vi "getStateValue.vi"(8 "error in (no error)":errorcluster, 11 "ScriptEvent in":refnum<class "ScriptEvent.lvclass">) -> (0 "error out":errorcluster, 2 "stateValue":string, 3 "ScriptEvent out":refnum<class "ScriptEvent.lvclass">)   [LabVIEW 2011, in "Tools.lvlib" / "Scripting.lvlib" / "ScriptEvent.lvclass"]
uses:
  ScriptEvent.lvclass
  ScriptEvent.lvclass/ScriptEvent.ctl
  DatabaseHelpers/Database Objects/Channel/Channel.lvclass
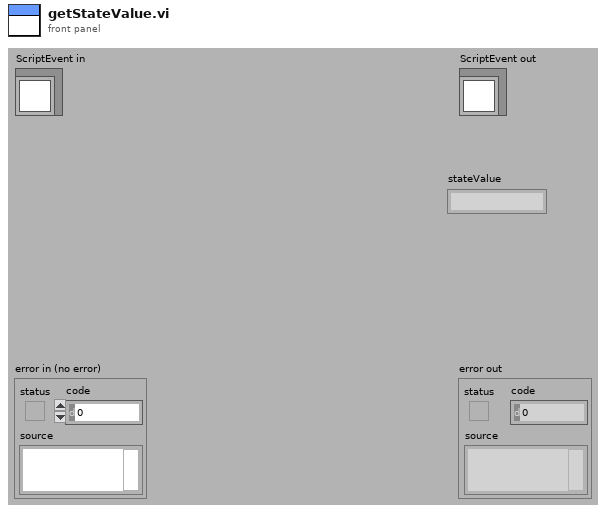
[diagram p1: front panel]
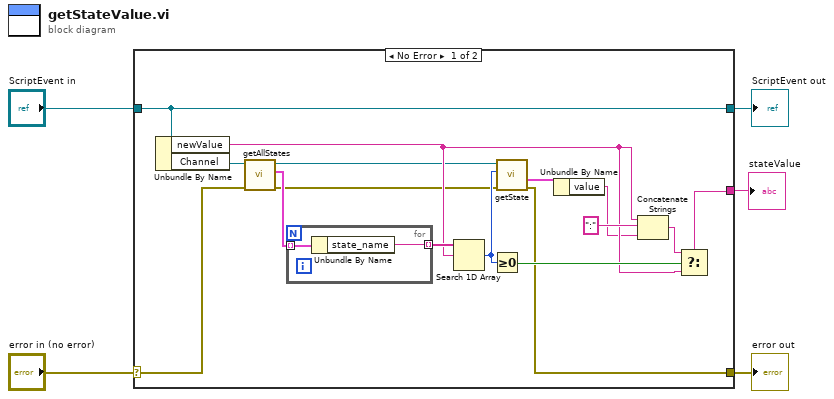
[diagram p0: block diagram]
diagram:
  n1 = case shown="No Error" "error in (no error)" {
    selector: "error in (no error)" -> [w10 w25]
    tunnel: [w6 w25] -> w4
    tunnel: [w21 w24] -> w2
    tunnel: "ScriptEvent in" -> [w21 w24]
    tunnel: [w7 _] -> w1
    frame No Error {
      n2 = Unbundle By Name(w21) -> ("newValue"=w14:string, "Channel"=w20:refnum<class "Channel.lvclass">)
      n3 = call "getAllStates.vi"("error in (no error)"=w10, "Channel.lvclass in"=w20) -> ("error out"=w11:errorcluster, "states"=w15:cluster{"state_name":string, "value":string}[], "Channel.lvclass out"=w13:refnum<class "Channel.lvclass">)  [unwired: 7 in]
      n4 = for {
        tunnel: w15 -> [w23] mode=indexing
        tunnel: [w22] -> w19 mode=indexing
        n5 = Unbundle By Name(w23) -> ("state_name"=w22:string)
      }
      n6 = Search 1D Array(1D array=w19, element=w14) -> (index of element=w12:i32)  [unwired: 1 in]
      n7 = Greater Or Equal To 0?(x=w12) -> (x >= 0?=w16:bool)
      n8 = call "getState.vi"("error in (no error)"=w11, "index"=w12, "Channel.lvclass in"=w13) -> ("error out"=w6:errorcluster, "state"=w9:cluster{"state_name":string, "value":string})  [unwired: 6 in, 1 out]
      n9 = Unbundle By Name(w9) -> ("value"=w8:string)
      n10 = Concatenate Strings(w14, ":", w8) -> (w17:string)
      n11 = Select(t=w17, s=w16, f=w14) -> (s? t:f=w7:string)
    }
    frame Error {
    }
  }
  "error out" <- w4
  "ScriptEvent out" <- w2
  "stateValue" <- w1
